vi "fgv_erp42mini-opval.vi"(7 "cmd":enum16{"ini", "read", "wirte"}(ring), 11 "car_v":T1 {"speed_curr" format="%1_1g"; "Dir" scale=0.0..2.0; "Brake" scale=0.0..200.0; "Steer_set" scale=-2000.0..2000.0; "Acc_set" scale=0.0..100.0}) -> (3 "car_v_out":T1)   [LabVIEW 2019]
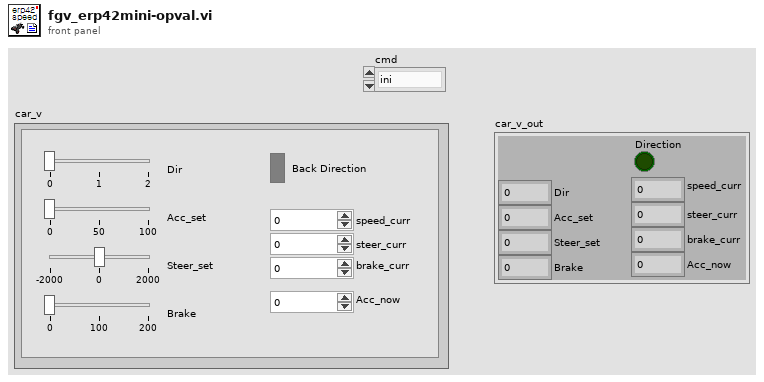
[diagram p1: front panel]
types:
  T1 = cluster{"Dir":u8, "Acc_set":u16, "Steer_set":i16, "Brake":i16, "Direction":bool, "speed_curr":dbl, "steer_curr":i16, "brake_curr":i16, "Acc_now":i16}
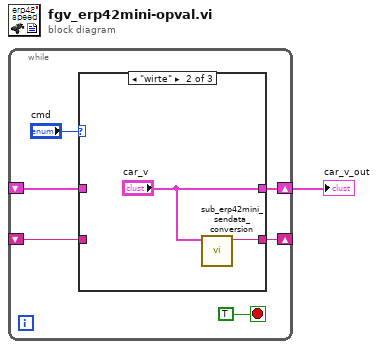
[diagram p0: block diagram]
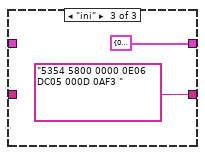
[diagram p3: hidden frame]
diagram:
  n1 = while {
    shift-right: [w5] -> w1
    shift-left: _ -> [w4]
    shift-right: [w3] -> _
    shift-left: _ -> [w2]
    stop <- TRUE stop-if-true
    n2 = case shown="\"wirte\"" "cmd" {
      tunnel: [w9 "car_v" T1 {"Dir"=0, "Acc_set"=0, "Steer_set"=0, "Brake"=0, "Direction"=FALSE, "speed_curr"=0.0, "steer_curr"=0, "brake_curr"=0, "Acc_now"=0} ("car_v")] -> w5
      tunnel: w4 -> [w9 _ _]
      tunnel: [w8 w10 "5354 5800 0000 0E06 DC05 000D 0AF3 " ("drive_v_strout")] -> w3
      tunnel: w2 -> [w8 _ _]
      frame "read", Default {
      }
      frame "wirte" {
        n3 = call "sub_erp42mini_sendata_conversion.vi"("car_v"="car_v") -> ("drive_v_strout"=w10:string)  [unwired: 10 in]
      }
      frame "ini" {
      }
    }
  }
  "car_v_out" <- w1
